vi "Main DMA FIFO test.vi"() -> ()   [LabVIEW 2019]
uses:
  <vilib>/Platform/TimedLoop/XDataNode/timing_clust.ctl
  <vilib>/Platform/TimedLoop/XDataNode/nitl_modes.ctl
  <vilib>/Platform/TimedLoop/XDataNode/wakeup.ctl
  <vilib>/rvi/Emulation/niFpgaSctlEmulationGetInTimedLoop.vi
  <vilib>/rvi/Emulation/niFpgaProcessEmulError.vi
  <vilib>/rvi/eio/common/nirviEmuTemplateMethod_errors.vi
  <vilib>/rvi/Emulation/niFpgaEmulationReportErrorSimple.vi
  <vilib>/rvi/Emulation/niFpgaGetClockAttributes.vi
  <vilib>/rvi/Emulation/niFpgaCriticalErrorInLSC.vi
  <vilib>/rvi/interface/RandomDataEmulation/niFpgaRandomDataHandleErrors.vi
  <vilib>/eio/EIONode/EIONode.xnode
  <vilib>/platform/TimedLoop/XDataNode/XDataNode.xnode
  <vilib>/rvi/DataTransferAndStorage/Container/XNode/niFpgaContainer.xnode
  <vilib>/rvi/interface/RandomDataEmulation/nirviRandomDataFpgaReadWriteTemplate.vi
  <vilib>/Platform/TimedLoop/XDataNode/XDNodeRunTimeDep.lvlib
panel:
  out "xt success":bool
  in  "GPIB0":u32
  in  "xt0":u32
  in  "xt total":u32
  in  "xt end":u32
  out "xt counter":u32
  out "elapsed":u32
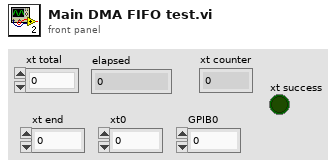
[diagram p1: front panel]
types:
  T1 = typedef "XDNodeRunTimeDep.lvlib/timing_clust.ctl" = cluster{"Expected End [f-1]":u64, "Actual End [f-1]":u64, "Finished Late? [f-1]":bool, "Expected End [i-1]":u64, "Actual End [i-1]":u64, "Finished Late? [i-1]":bool, "Expected Start [i]":u64, "Actual Start [i]":u64, "Expected Start [f]":u64, "Actual Start [f]":u64, "Source Name":string, "Structure Name":string, "Period":i64, "Deadline":i64, "Offset":i64, "Start":i64, "Priority":i32, "Timeout":i32, "Mode":T2, "Wakeup Reason":T3, "Error":errorcluster, "Source Type":string, "Secondary Source Type":string, "Global End Time":u64, "Global Start Time":u64, "Frame Duration":u64, "Iteration Duration":u64, "Assigned CPU":i32, "I/O Scan Engine Mode":u32}
  T2 = typedef "XDNodeRunTimeDep.lvlib/nitl_modes.ctl" = enum32{"No Change", "Process missed periods, maintain original phase", "Discard missed periods, maintain original phase", "Process missed periods, ignore original phase", "Discard missed periods, ignore original phase"}
  T3 = typedef "XDNodeRunTimeDep.lvlib/wakeup.ctl" = enum32{"Normal", "Aborted", "Asynchronous wakeup", "Timing source error", "Timed loop error", "Timeout"}
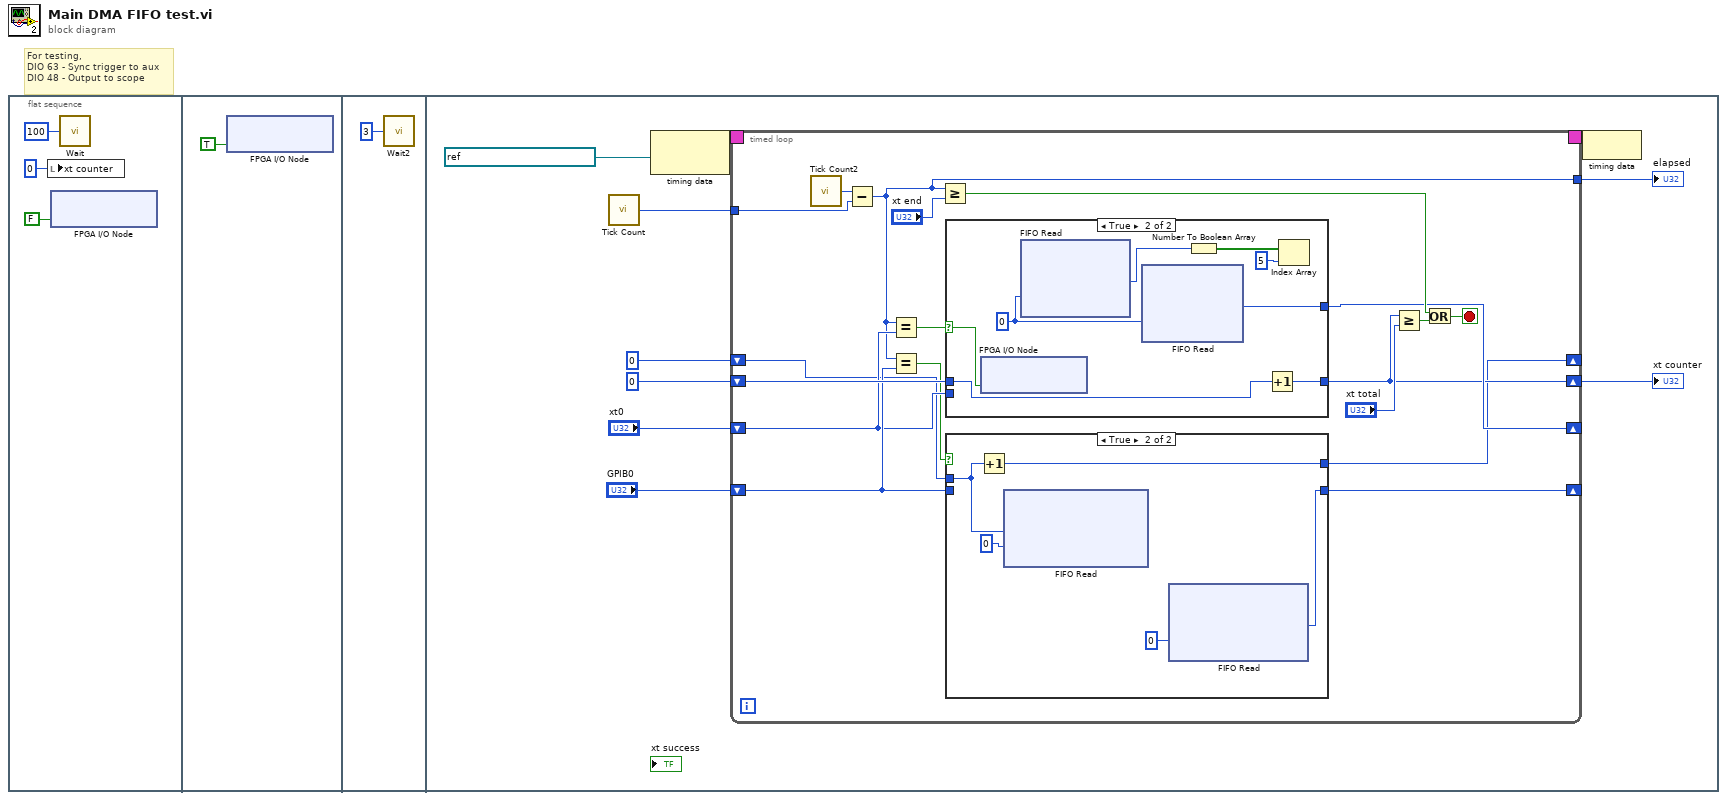
[diagram p0: block diagram]
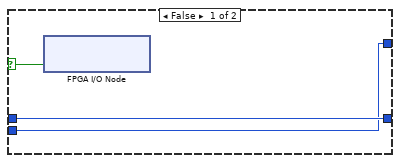
[diagram p3: hidden frame]
diagram:
  # "For testing,\nDIO 63 - Sync trigger to aux\nDIO 48 - Output to scope"
  n1 = flat-sequence {
    frame #0 {
      n2 = local write "xt counter"(u32 0 ("xt counter")) -> ()
      n3 = xnode "FPGA I/O Node"("RMC/DIO63"=FALSE) -> ()  [unwired: 1 in, 1 out]
      n4 = call "Wait"("Count(mSec)"=u8 100) -> ()  [unwired: 1 out]
    }
    frame #1 {
      n5 = xnode "FPGA I/O Node"("RMC/DIO63"=TRUE) -> ()  [unwired: 1 in, 1 out]
    }
    frame #2 {
      n6 = call "Wait2"("Count(Ticks)"=u8 3) -> ()  [unwired: 1 out]
    }
    frame #3 {
      n7 = call "Tick Count"() -> ("Tick Count(uSec)"=w15:u32)
      n8 = node-c288(refnum<k21> "40 MHz Onboard Clock" ("Source Name")) -> (w9:T1)
      n9 = timed-loop {
        tunnel: w15 -> [w32]
        shift-right: [w22] -> w12
        shift-left: u32 0 ("xt counter") -> [w33]
        shift-right: [w25] -> _
        shift-left: "xt0" -> [w26]
        shift-right: [w30] -> _
        shift-left: "GPIB0" -> [w31]
        tunnel: [w18] -> w13
        timing: w9 -> [_]
        timing-out: [_] -> w8
        shift-right: [w16] -> _
        shift-left: u16 0 -> [w17]
        stop <- w28 stop-if-true
        n10 = call "Tick Count2"() -> ("Tick Count(uSec)"=w21:u32)
        n11 = Subtract(x=w21, y=w32) -> (x-y=w18:u32)
        n12 = Equal?(x=w18, y=w26) -> (x = y?=w20:bool)
        n13 = Equal?(x=w18, y=w31) -> (x = y?=w19:bool)
        n14 = Greater Or Equal?(x=w18, y="xt end") -> (x >= y?=w29:bool)
        n15 = case shown="True" w20 {
          selector: w20 -> [w41 w45]
          tunnel: [w42 w51] -> w25
          tunnel: [w43 w48] -> w22
          tunnel: w33 -> [w43 w47]
          tunnel: w26 -> [w42 _]
          frame False {
            n16 = xnode "FPGA I/O Node"("RMC/DIO48"=w41) -> ()  [unwired: 1 in, 1 out]
          }
          frame True {
            w46 = 0 ("index")
            n17 = xnode "FPGA I/O Node"("RMC/DIO48"=w45) -> ()  [unwired: 1 in, 1 out]
            n18 = xnode ("FIFO Read")("Timeout"=w46) -> ("Element"=w44:u32)  [unwired: 1 in, 2 out]
            n19 = xnode ("FIFO Read")("Timeout"=w46) -> ("Element"=w51:u32)  [unwired: 1 in, 2 out]
            n20 = Number To Boolean Array(number=w44) -> (Boolean array=w50:bool[])
            n21 = Increment(x=w47) -> (x+1=w48:u32)
            n22 = Index Array(array=w50, index=5) -> ()  [unwired: 1 out]
          }
        }
        n23 = case shown="True" w19 {
          tunnel: w31 -> [w35 _]
          tunnel: [w35 w39] -> w30
          tunnel: w17 -> [w34 w37]
          tunnel: [w34 w36] -> w16
          frame False {
          }
          frame True {
            n24 = Increment(x=w37) -> (x+1=w36:u16)
            n25 = xnode ("FIFO Read")("Element"=w37, "Timeout"=u8 0) -> ()  [unwired: 1 in, 2 out]
            n26 = xnode ("FIFO Read")("Timeout"=0) -> ("Element"=w39:u32)  [unwired: 1 in, 2 out]
          }
        }
        n27 = Greater Or Equal?(x=w22, y="xt total") -> (x >= y?=w24:bool)
        n28 = Or(x=w29, y=w24) -> (x .or. y?=w28:bool)
      }
      "elapsed" <- w13
      "xt counter" <- w12
      n29 = node-c288(w8) -> ()
    }
  }
